vi "Write Event Type.vi"(8 "error in (no error)":errorcluster, 10 "Event Type (New)":T1, 11 "VI in":refnum<class "VI.lvclass">) -> (0 "error out":errorcluster, 3 "VI out":refnum<class "VI.lvclass">)   [LabVIEW 2019, in "Panther Dashboard.lvlib" / "VI.lvclass"]
uses:
  VI.lvclass
  <vilib>/Delacor/Delacor QMH/Libraries/_Scripting Support/Event Type (New)--enum.ctl
  VI.lvclass/VI.ctl
  <vilib>/Delacor/Delacor QMH/Libraries/_Scripting Support/dqmh_lib_DQMH Scripting Support.lvlib
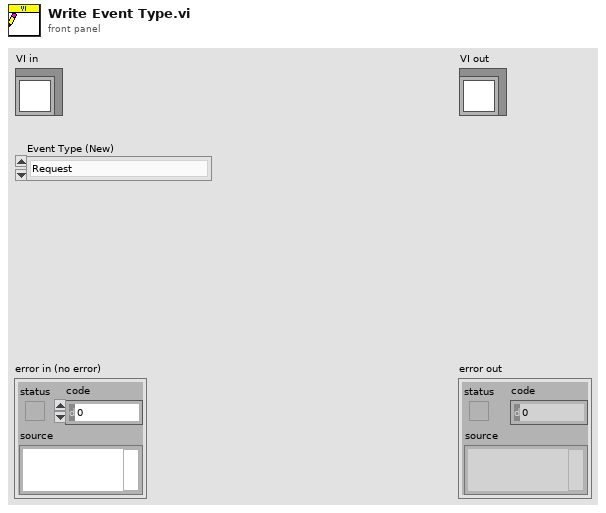
[diagram p1: front panel]
types:
  T1 = typedef "dqmh_lib_DQMH Scripting Support.lvlib/Event Type (New)--enum.ctl" = enum16{"Request", "Broadcast", "Request and Wait for Reply", "Round Trip"}
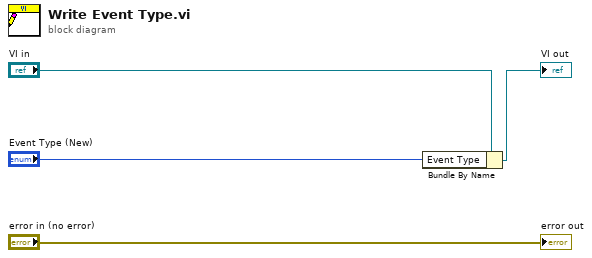
[diagram p0: block diagram]
diagram:
  n1 = Bundle By Name(cluster="VI in", "Event Type"="Event Type (New)") -> (→"VI out":refnum<class "VI.lvclass">)
  "error out" <- "error in (no error)"
